vi "Objective_init.vi"(8 "error in (no error)":errorcluster, 10 "maxEval":dbl, 11 "Objective in":refnum<class "Objective.lvclass">) -> (0 "error out":errorcluster, 3 "Objective out":refnum<class "Objective.lvclass">)   [LabVIEW 2023, in "Objective.lvclass"]
uses:
  Objective.lvclass
  Objective.lvclass/Objective.ctl
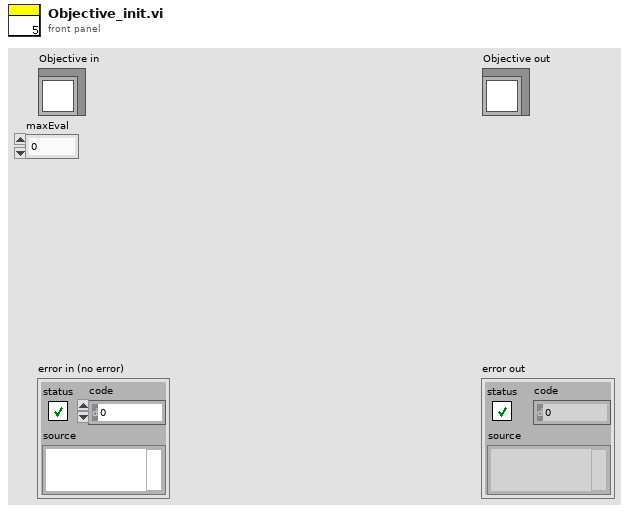
[diagram p1: front panel]
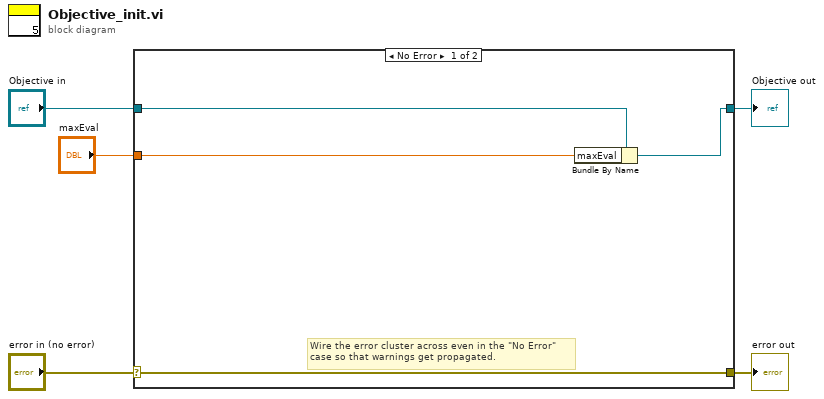
[diagram p0: block diagram]
diagram:
  n1 = case shown="No Error" "error in (no error)" {
    selector: "error in (no error)" -> [w9 w11]
    tunnel: [w9 w11] -> w4
    tunnel: [w7 w10] -> w2
    tunnel: "Objective in" -> [w8 w10]
    tunnel: "maxEval" -> [w6 _]
    frame No Error {
      # "Wire the error cluster across even in the \"No Error\"\ncase so that warnings get propagated."
      n2 = Bundle By Name(cluster=w8, "maxEval"=w6) -> (w7:refnum<class "Objective.lvclass">)
    }
    frame Error {
    }
  }
  "error out" <- w4
  "Objective out" <- w2
